vi "Cleanup client and server backup.vi"(8 "error in":errorcluster, 10 "Revert":bool, 11 "proto File Path":path) -> (0 "error out":errorcluster)   [LabVIEW 2021, in "TemplateCoreUtilities.lvlib"]
uses:
  TemplateCoreUtilities.lvlib
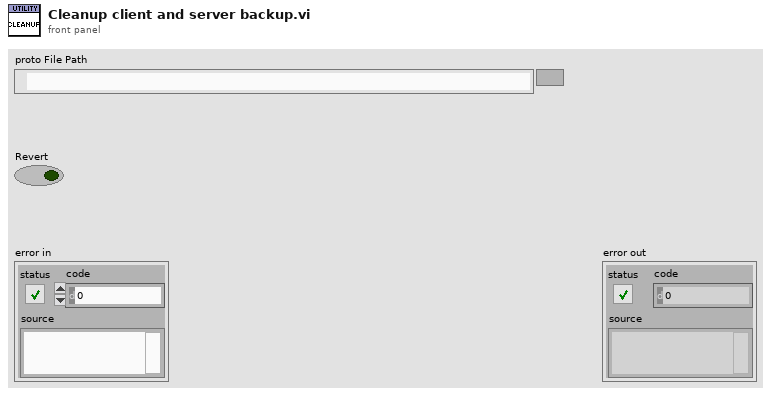
[diagram p1: front panel]
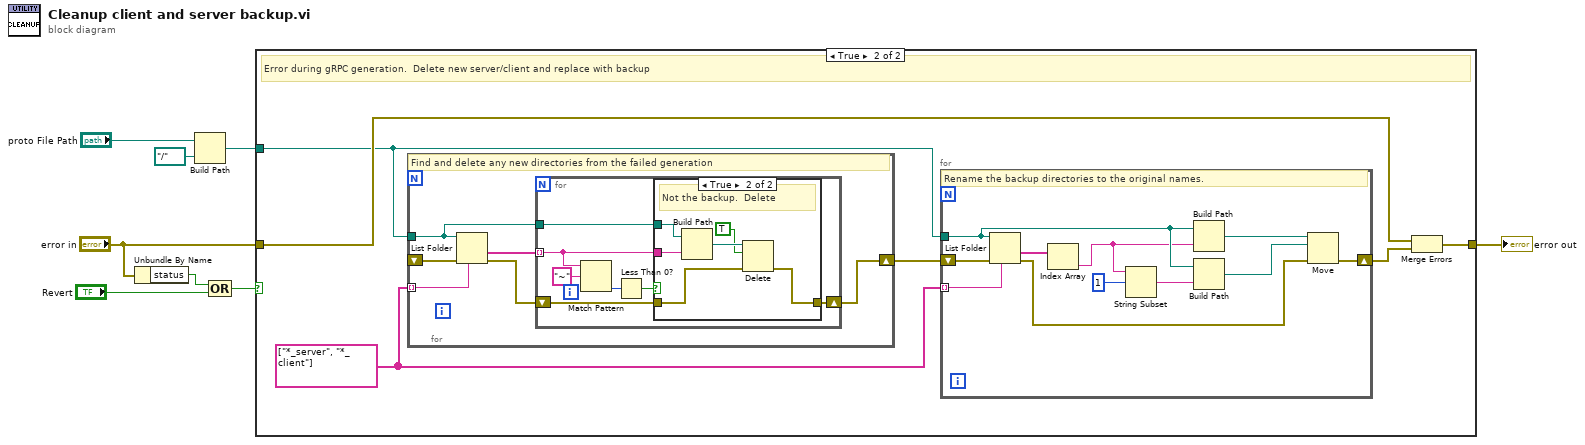
[diagram p0: block diagram]
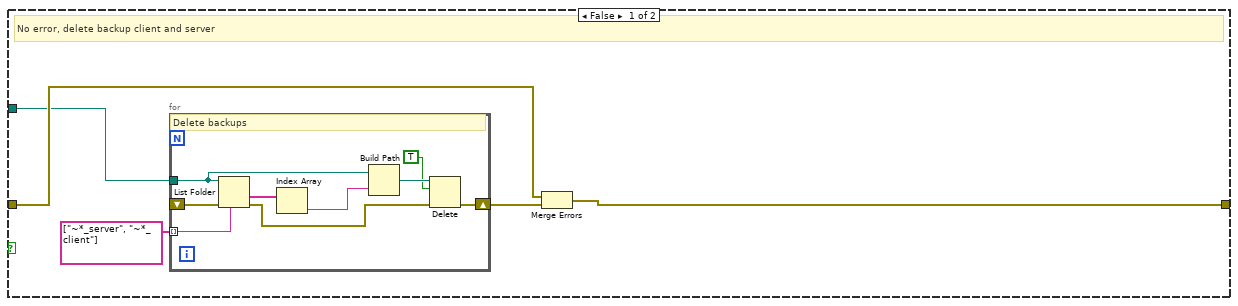
[diagram p2: hidden frame]
diagram:
  n1 = Unbundle By Name("error in") -> ("status"=w7:bool)
  n2 = Build Path(base path="proto File Path", name or relative path=path "../..") -> (appended path=w1:path)
  n3 = Compound Arithmetic op=OR(w7, "Revert") -> (w6:bool)
  n4 = case shown="True" w6 {
    tunnel: [w10 w26] -> w8
    tunnel: w1 -> [w9 w23]
    tunnel: "error in" -> [w11 w24]
    frame False {
      # "No error, delete backup client and server"
      n5 = for {
        tunnel: w9 -> [w19]
        tunnel: string[] ["~*_server", "~*_client"] -> [w21] mode=indexing
        shift-right: [w15] -> w12
        shift-left: _ -> [w20]
        # "Delete backups"
        n6 = List Folder(path=w19, pattern=w21, error in=w20) -> (folder names=w22:string[], error out=w16:errorcluster)  [unwired: 1 in, 2 out]
        n7 = Index Array(array=w22) -> (element=w18:string)  [unwired: 1 in]
        n8 = Build Path(base path=w19, name or relative path=w18) -> (appended path=w17:path)
        n9 = Delete(path (use dialog)=w17, entire hierarchy (F)=TRUE, error in=w16) -> (error out=w15:errorcluster)  [unwired: 2 in, 2 out]
      }
      n10 = Merge Errors(w11, w12) -> (w10:errorcluster)
    }
    frame True {
      w27 = string[] ["*_server", "*_client"]
      # "Error during gRPC generation.  Delete new server/client and replace with backup"
      n11 = for {
        tunnel: w23 -> [w43]
        tunnel: w27 -> [w45] mode=indexing
        shift-right: [w41] -> w28
        shift-left: _ -> [w44]
        # "Find and delete any new directories from the failed generation"
        n12 = List Folder(path=w43, pattern=w45, error in=w44) -> (folder names=w40:string[], error out=w42:errorcluster)  [unwired: 1 in, 2 out]
        n13 = for {
          tunnel: w43 -> [w52]
          shift-right: [w50] -> w41
          shift-left: w42 -> [w51]
          tunnel: w40 -> [w46] mode=indexing
          n14 = Match Pattern(string=w46, regular expression="~") -> (offset past match=w48:i32)  [unwired: 1 in, 3 out]
          n15 = Less Than 0?(x=w48) -> (x < 0?=w47:bool)
          n16 = case shown="True" w47 {
            tunnel: w52 -> [_ w59]
            tunnel: w51 -> [w53 w57]
            tunnel: [w53 w56] -> w50
            tunnel: w46 -> [_ w55]
            frame False {
              # "Backup.  Do nothing"
            }
            frame True {
              # "Not the backup.  Delete"
              n17 = Build Path(base path=w59, name or relative path=w55) -> (appended path=w58:path)
              n18 = Delete(path (use dialog)=w58, entire hierarchy (F)=TRUE, error in=w57) -> (error out=w56:errorcluster)  [unwired: 2 in, 2 out]
            }
          }
        }
      }
      n19 = for {
        tunnel: w23 -> [w37]
        tunnel: w27 -> [w34] mode=indexing
        shift-right: [w32] -> w25
        shift-left: w28 -> [w33]
        # "Rename the backup directories to the original names."
        n20 = List Folder(path=w37, pattern=w34, error in=w33) -> (folder names=w39:string[], error out=w35:errorcluster)  [unwired: 1 in, 2 out]
        n21 = Index Array(array=w39) -> (element=w31:string)  [unwired: 1 in]
        n22 = String Subset(string=w31, offset (0)=1) -> (substring=w30:string)  [unwired: 1 in]
        n23 = Build Path(base path=w37, name or relative path=w31) -> (appended path=w38:path)
        n24 = Build Path(base path=w37, name or relative path=w30) -> (appended path=w36:path)
        n25 = Move(source path=w38, error in=w35, 10:w36) -> (error out=w32:errorcluster)  [unwired: 2 in, 2 out]
      }
      n26 = Merge Errors(w24, w25) -> (w26:errorcluster)
    }
  }
  "error out" <- w8
